vi "ATSh_GetChannelnfo.vi"(11 "HandleIn":u32) -> (0 "Return Code":u32, 1 "SampleSize":u8, 2 "MemSize/Channel(Sample)":u32, 3 "HandleOut":u32, 4 "MaxPretriggerSamples":u32)   [LabVIEW 2010]
doc: "_____AlazarTech, Scope_____\n\nRetrieve channel memory size as well as the sample size and the Maximum available Pretrigger Samples."
uses:
  ATS_ctl/ATS_Query.ctl
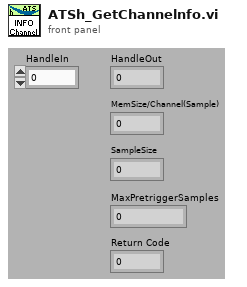
[diagram p1: front panel]
types:
  T1 = typedef "ATS_Query.ctl" = enum16{"None", "NUMBER_OF_RECORDS", "PRETRIGGER_AMOUNT", "RECORD_LENGTH", "TRIGGER_ENGINE", "TRIGGER_DELAY", "TRIGGER_TIMEOUT", "SAMPLE_RATE", "CONFIGURATION_MODE", "DATA_WIDTH", "AUTO_CALIBRATE", "TRIGGER_XXXXX", "CLOCK_SOURCE", "CLOCK_SLOPE", "IMPEDANCE", "INPUT_RANGE", "COUPLING", "MAX_TIMEOUTS_ALLOWED", "ATS_OPERATING_MODE", "CLOCK_DECIMATION_EXTERNAL", "LED_CONTROL", "ATTENUATOR_RELAY", "EXT_TRIGGER_COUPLING", "EXT_TRIGGER_ATTENUATOR_RELAY", "TRIGGER_ENGINE_SOURCE", "TRIGGER_ENGINE_SLOPE", "SEND_DAC_VALUE", "SLEEP_DEVICE", "MEMORY_SIZE", "BOARD_TYPE", "ASOPC_TYPE", "SERIAL_NUMBER", "FIRSTCAL_DATE", "LATEST_CAL_DATE", "LATEST_TEST_DATE"}
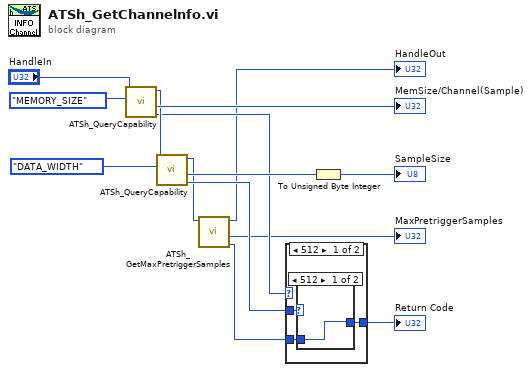
[diagram p0: block diagram]
diagram:
  n1 = call "ATSh_QueryCapability.vi"("ATS_Query"=ATS_Query."MEMORY_SIZE", "HandleIn"="HandleIn") -> ("Return Code"=w8:u32, "ReturnValue"=→"MemSize/Channel(Sample)":u32, "HandleOut"=w11:u32)  [unwired: 6 in, 1 out]
  n2 = call "ATSh_QueryCapability.vi"("ATS_Query"=ATS_Query."DATA_WIDTH", "HandleIn"=w11) -> ("Return Code"=w7:u32, "ReturnValue"=w12:u32, "HandleOut"=w5:u32)  [unwired: 6 in, 1 out]
  n3 = call "ATSh_GetMaxPretriggerSamples.vi"("HandleIn"=w5) -> ("Return Code"=w2:u32, "MaxPretriggerSamples"=→"MaxPretriggerSamples":u32, "HandleOut"=→"HandleOut":u32)  [unwired: 8 in]
  n4 = case shown="512" w8 {
    selector: w8 -> [_ w20]
    tunnel: w7 -> [w17 _]
    tunnel: [w16 w20] -> w6
    tunnel: w2 -> [w15 _]
    frame 512 {
      n5 = case shown="512" w17 {
        selector: w17 -> [_ w19]
        tunnel: w15 -> [w18 _]
        tunnel: [w18 w19] -> w16
        frame 512 {
        }
        frame 1, Default {
        }
      }
    }
    frame 1, Default {
    }
  }
  "Return Code" <- w6
  n6 = To Unsigned Byte Integer(number=w12) -> (unsigned 8bit integer=→"SampleSize":u8)
